vi "Pcre2SubstringCopyByName8.vi"(8 "error in":errorcluster, 10 "Name":string, 11 "pMatchData":u64 format="%.0x") -> (0 "error out":errorcluster, 2 "Substring":string, 3 "pMatchData":u64 format="%.0x")   [LabVIEW 2021, in "libpcre2-8.lvlib"]
uses:
  libpcre2-8.lvlib
  libpcre2-8-x32.dll
panel:
  in  "Length":u64
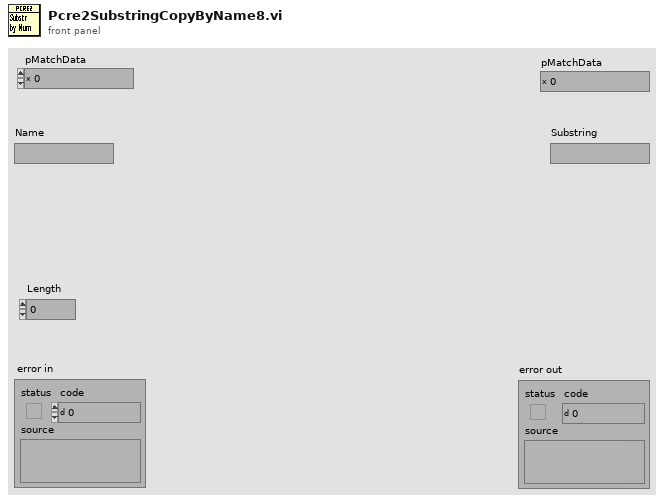
[diagram p1: front panel]
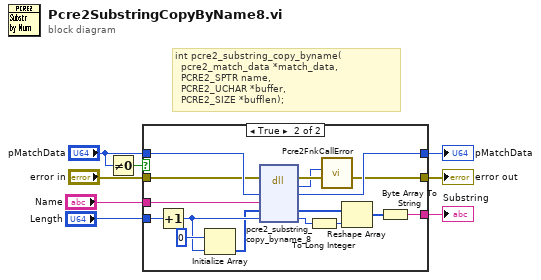
[diagram p0: block diagram]
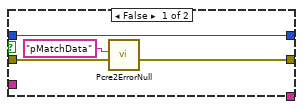
[diagram p2: hidden frame]
diagram:
  # "int pcre2_substring_copy_byname(\n  pcre2_match_data *match_data,\n  PCRE2_SPTR name,\n  PCRE2_UCHAR *buffer,\n  PCRE2_SIZE *bufflen);"
  n1 = Not Equal To 0?(x="pMatchData") -> (x != 0?=w5:bool)
  n2 = case shown="True" w5 {
    tunnel: "error in" -> [w11 w17]
    tunnel: [w10 w26] -> w7
    tunnel: "pMatchData" -> [w12 w18]
    tunnel: [w12 w28] -> w6
    tunnel: [_ w23] -> w2
    tunnel: "Name" -> [_ w24]
    tunnel: "Length" -> [_ w16]
    frame False {
      n3 = call "Pcre2ErrorNull.vi"("error in"=w11, "What"="pMatchData" ("message")) -> ("error out"=w10:errorcluster)  [unwired: 9 in]
    }
    frame True {
      n4 = Increment(x=w16) -> (x+1=w14:u64)
      n5 = Initialize Array(u8 0 ("U8"), w14) -> (w13:u8[])
      n6 = dll-call lib="libpcre2-8-x*.dll" fn="pcre2_substring_copy_byname_8"(error in=w17, "match_data"=w18, "name"=w24, "buffer"=w13, "bufflen"=w14) -> (error out=w27:errorcluster, "return type"=w25:i32, "match_data"=w28:u64, "buffer"=w22:u8[], "bufflen"=w20:u64)  [unwired: 3 in, 1 out]
      n7 = To Long Integer(number=w20) -> (32bit integer=w19:i32)
      n8 = call "Pcre2FnkCallError.vi"("error in"=w27, "ErrorCode"=w25) -> ("error out"=w26:errorcluster)  [unwired: 9 in]
      n9 = Reshape Array(w22, w19) -> (w21:u8[])
      n10 = Byte Array To String(unsigned byte array=w21) -> (string=w23:string)
    }
  }
  "pMatchData" <- w6
  "error out" <- w7
  "Substring" <- w2
